vi "CALC_DATA_SNP_PORT_SAVE.vi"(0 "VISA IN":refnum<visa-resource-name>, 1 "Port numbers":string, 2 "File Path":string, 5 "error in":errorcluster, 7 "Channel":i32) -> (14 "VISA Out":refnum<visa-resource-name>, 19 "error out":errorcluster)   [LabVIEW 2018, in "PNA-X.lvlib"]
doc: "CALCulate<cnum>:DATA:SNP:PORTs:SAVE <\"x,y,z\">,<filename> \nNote: This command replaces MMEM:STOR sNp. This command is more explicit regarding the data \nto be saved, and works for PNAs with multiport test sets. \n(Write-only) Saves sNp data from the selected measurement for the specified ports. \nLearn more about SNP data. \nSee Critical Note \nParameters \n<cnum> Channel number of the measurement. There must be a selected measurement \non that channel. If unspecified, <cnum> is set to 1. \n<\"x,y,z\"> String Comma or space delimited port numbers for which data is requested, \nenclosed in quotes. \n<filename> String Path, filename, and suffix of location to store the sNp data. The suffix \nis not checked for accuracy. If saving 2 ports, specify \"filename.s2p\"; If saving \n4 ports, specify \"filename.s4p.\", and so forth. \nSnP data can be output using several data formatting options. See \nMMEM:STORe:TRACe:FORMat:SNP. \nExamples CALC:DATA:SNP:PORTs:Save '1,2,4','C:/Program \nFiles/Agilent/Network Analyzer/Documents/MyData.s3p' \nReturn Type Depends on FORMat:DATA \nDefault Not Applicable \nLast modified: \nApril 26, 2007 Added clarification to Calc:Data SDATA \n9/18/06 MQ Added two SNP Ports commands for multiport \n1502\n\nCalculate:Equation Commands \nControls Equation Editor capabilities. \nClick on a blue keyword to view the command details. \nSee Also \nExample Programs \nLearn about Equation Editor \nSynchronizing the PNA and Controller \nSCPI Command Tree \nCritical Note: CALCulate commands act on the selected measurement. You can select one \nmeasurement for each channel using Calc:Par:Select"
uses:
  PNA-X.lvlib
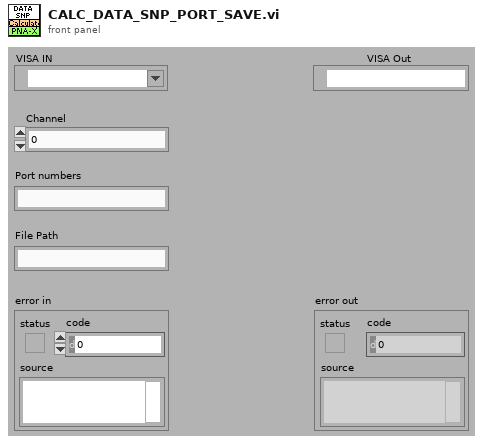
[diagram p1: front panel]
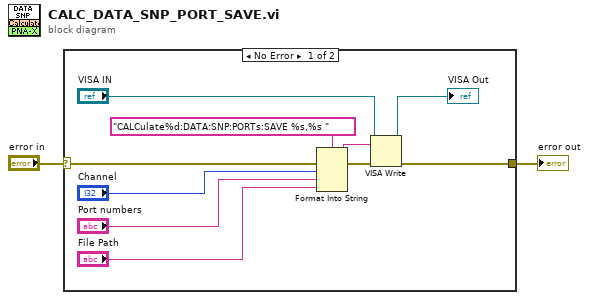
[diagram p0: block diagram]
diagram:
  n1 = case shown="No Error" "error in" {
    selector: "error in" -> [w12 w13]
    tunnel: [w7 w13] -> w1
    frame No Error {
      n2 = Format Into String(format string="CALCulate%d:DATA:SNP:PORTs:SAVE %s,%s " ("Cmdline"), error in=w12, "Channel", "Port numbers", "File Path") -> (resulting string=w10:string, error out=w11:errorcluster)  [unwired: 1 in]
      n3 = VISA Write(VISA resource name="VISA IN", write buffer=w10, error in (no error)=w11) -> (VISA resource name out=→"VISA Out":refnum<visa-resource-name>, error out=w7:errorcluster)  [unwired: 1 out]
    }
    frame Error {
    }
  }
  "error out" <- w1
